vi "writeToCommandValve00.vi"(1 "error in (no error)":errorcluster, 2 "delay (ms) 2":u32=200, 3 "String":string) -> (0 "error out":errorcluster)   [LabVIEW 2011]
panel:
  in  "delay (ms)":u32=200
  out "concatenated string":string
  out "VISA resource name out":refnum<visa-resource-name>
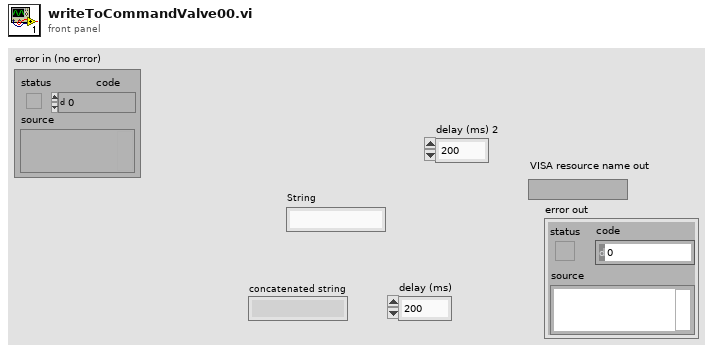
[diagram p1: front panel]
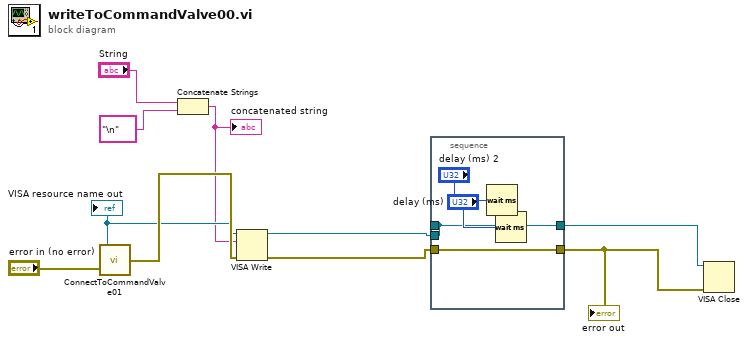
[diagram p0: block diagram]
diagram:
  n1 = call "ConnectToCommandValve01.vi"("error in (no error)"="error in (no error)") -> ("error out"=w10:errorcluster, "VISA resource name out"=w9:refnum<visa-resource-name>)
  "VISA resource name out" <- w9
  n2 = Concatenate Strings("String", "\n") -> (w7:string)
  "concatenated string" <- w7
  n3 = VISA Write(VISA resource name=w9, write buffer=w7, error in (no error)=w10) -> (VISA resource name out=w2:refnum<visa-resource-name>, error out=w3:errorcluster)  [unwired: 1 out]
  n4 = stacked-sequence {
    tunnel: w3 -> [w14]
    tunnel: [w14] -> w5
    tunnel: [w12] -> _
    tunnel: [w12] -> w4
    tunnel: w2 -> [w12]
    frame #0 {
      n5 = Wait (ms)(milliseconds to wait="delay (ms) 2") -> ()  [unwired: 1 out]
    }
  }
  "error out" <- w5
  n6 = Wait (ms)(milliseconds to wait="delay (ms)") -> ()  [unwired: 1 out]
  n7 = VISA Close(VISA resource name=w4, error in (no error)=w5) -> ()  [unwired: 1 out]
